vi "Detecting 0rpm.vi"(8 "error in":errorcluster, 10 "RPM":dbl) -> (0 "error out":errorcluster)   [LabVIEW 2020, in "Cycling by Event module.lvlib"]
doc: "When 0rpm reaching, change state to \"Accelerating to 110rpm\" in helper loop for next cycle\n_____\nCreated using DQMH Event Scripter 7.0.1.1316."
uses:
  Cycling by Event module.lvlib
  Detecting 0rpm Argument--cluster.ctl
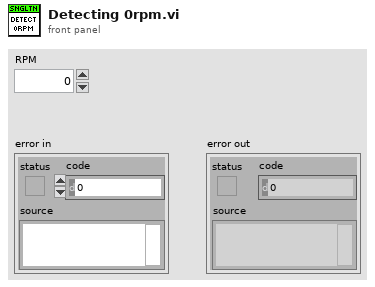
[diagram p1: front panel]
types:
  T1 = typedef "Cycling by Event module.lvlib/Detecting 0rpm Argument--cluster.ctl" = cluster{"RPM":dbl}
  T2 = typedef "Cycling by Event module.lvlib/Request Events--cluster.ctl" = cluster{"Stop Module":refnum<user-event>, "Show Panel":refnum<user-event>, "Hide Panel":refnum<user-event>, "Get Module Execution Status":refnum<user-event>, "Show Diagram":refnum<user-event>, "Start cycling":refnum<user-event>, "Detecting 110rpm":refnum<user-event>, "Change state to HL":refnum<user-event>, "Detecting 100rpm":refnum<user-event>, "Detecting 0rpm":refnum<user-event>}
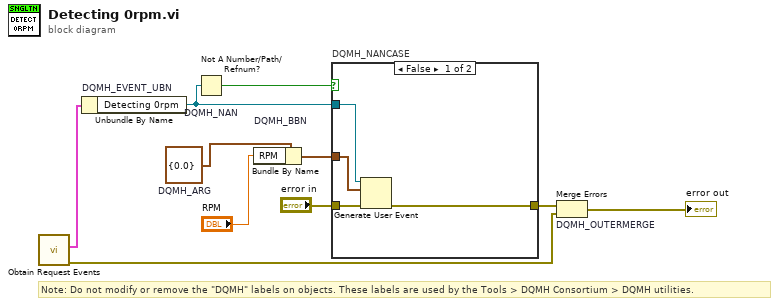
[diagram p0: block diagram]
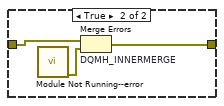
[diagram p2: hidden frame]
diagram:
  w4 = T1 {"RPM"=0.0}  # DQMH_ARG
  # "Note: Do not modify or remove the \"DQMH\" labels on objects. These labels are used by the Tools > DQMH Consortium > DQMH utilities."
  n1 = call "Obtain Request Events.vi"() -> ("error out"=w2:errorcluster, "Cycling by Event module Request Events"=w1:T2)  [unwired: 10 in]
  n2 = Unbundle By Name "DQMH_EVENT_UBN"(w1) -> ("Detecting 0rpm"=w6:refnum<user-event>)
  n3 = Not A Number/Path/Refnum? "DQMH_NAN"(number/path/refnum=w6) -> (NaN/Path/Refnum?=w7:bool)
  n4 = Bundle By Name "DQMH_BBN"(cluster=w4, "RPM"="RPM") -> (w8:T1)
  n5 = case "DQMH_NANCASE" shown="False" w7 {
    tunnel: "error in" -> [w14 w17]
    tunnel: [w13 w16] -> w5
    tunnel: w6 -> [w12 _]
    tunnel: w8 -> [w11 _]
    frame False {
      n6 = Generate User Event(user event=w12, event data cluster=w11, error in=w14) -> (error out=w13:errorcluster)  [unwired: 1 in, 1 out]
    }
    frame True {
      n7 = call "Module Not Running--error.vi"() -> ("error out"=w15:errorcluster)  [unwired: 11 in]
      n8 = Merge Errors "DQMH_INNERMERGE"(w17, w15) -> (w16:errorcluster)
    }
  }
  n9 = Merge Errors "DQMH_OUTERMERGE"(w5, w2) -> (→"error out":errorcluster)
